vi "github_tags.vi"() -> ()   [LabVIEW 2016]
panel:
  in  "version":string
  in  "commit":string
  in  "package":string
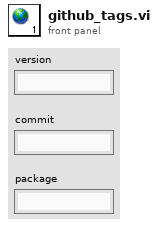
[diagram p1: front panel]
diagram:
